vi "DC_OUTPUT.vi"(1 "INPUT":T1) -> (0 "OUTPUT":T2)   [LabVIEW 2013]
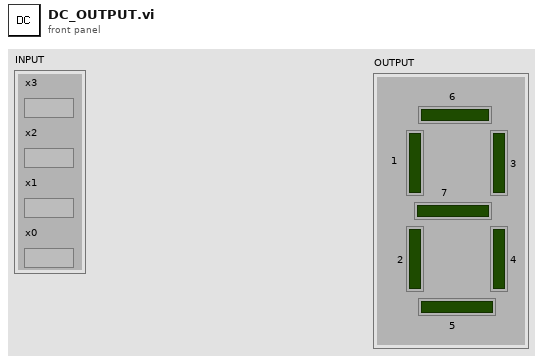
[diagram p1: front panel]
types:
  T1 = cluster{"x3":bool, "x2":bool, "x1":bool, "x0":bool}
  T2 = cluster{"6":bool, "3":bool, "1":bool, "7":bool, "2":bool, "4":bool, "5":bool}
  T3 = cluster{bool, bool, bool, bool, bool, bool, bool}
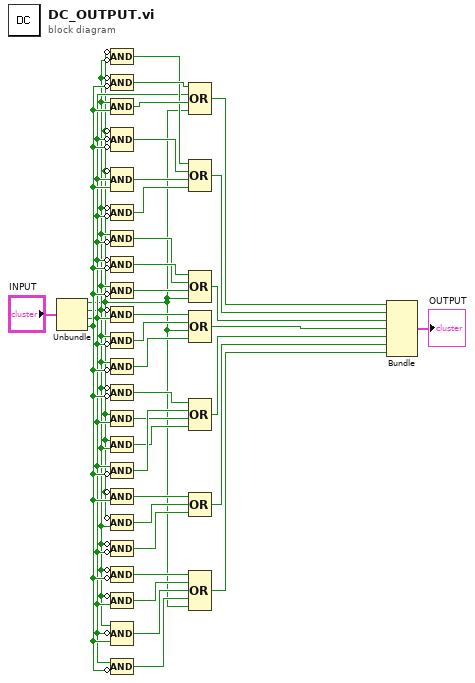
[diagram p0: block diagram]
diagram:
  n1 = Unbundle("INPUT") -> ("x3"=w1:bool, "x2"=w2:bool, "x1"=w3:bool, "x0"=w4:bool)
  n2 = Compound Arithmetic op=AND(invert w1, invert w2) -> (w34:bool)
  n3 = Compound Arithmetic op=AND(invert w2, invert w4) -> (w36:bool)
  n4 = Compound Arithmetic op=AND(w2, w4) -> (w35:bool)
  n5 = Compound Arithmetic op=AND(invert w1, invert w3, invert w4) -> (w33:bool)
  n6 = Compound Arithmetic op=AND(invert w1, w3, w4) -> (w32:bool)
  n7 = Compound Arithmetic op=AND(invert w2, invert w3) -> (w16:bool)
  n8 = Compound Arithmetic op=AND(w2, invert w3) -> (w30:bool)
  n9 = Compound Arithmetic op=AND(invert w3, invert w4) -> (w31:bool)
  n10 = Compound Arithmetic op=AND(w2, invert w4) -> (w29:bool)
  n11 = Compound Arithmetic op=AND(invert w2, w3) -> (w28:bool)
  n12 = Compound Arithmetic op=AND(w2, invert w3) -> (w27:bool)
  n13 = Compound Arithmetic op=AND(w2, invert w4) -> (w26:bool)
  n14 = Compound Arithmetic op=AND(invert w2, invert w4) -> (w25:bool)
  n15 = Compound Arithmetic op=AND(w1, w3) -> (w15:bool)
  n16 = Compound Arithmetic op=AND(w1, w2) -> (w14:bool)
  n17 = Compound Arithmetic op=AND(w3, invert w4) -> (w24:bool)
  n18 = Compound Arithmetic op=AND(invert w1, w4) -> (w23:bool)
  n19 = Compound Arithmetic op=AND(invert w1, w2) -> (w22:bool)
  n20 = Compound Arithmetic op=AND(invert w2, invert w3) -> (w21:bool)
  n21 = Compound Arithmetic op=AND(invert w2, invert w4) -> (w20:bool)
  n22 = Compound Arithmetic op=AND(invert w2, w3) -> (w19:bool)
  n23 = Compound Arithmetic op=AND(w2, invert w3, w4) -> (w18:bool)
  n24 = Compound Arithmetic op=AND(w3, invert w4) -> (w17:bool)
  n25 = Compound Arithmetic op=OR(w36, w3, w35, w1) -> (w13:bool)
  n26 = Compound Arithmetic op=OR(w34, w33, w32, w16) -> (w12:bool)
  n27 = Compound Arithmetic op=OR(w31, w30, w29, w1) -> (w11:bool)
  n28 = Compound Arithmetic op=OR(w28, w27, w1, w26) -> (w10:bool)
  n29 = Compound Arithmetic op=OR(w25, w24, w15, w14) -> (w9:bool)
  n30 = Compound Arithmetic op=OR(w23, w22, w21) -> (w8:bool)
  n31 = Compound Arithmetic op=OR(w20, w19, w18, w17, w1) -> (w7:bool)
  n32 = Bundle(w13, w12, w11, w10, w9, w8, w7) -> (→"OUTPUT":T3)  [unwired: 1 in]
